vi "Drive Process.vi"(0 "error in":errorcluster) -> ()   [LabVIEW 2013]
uses:
  Drive Global Data.vi
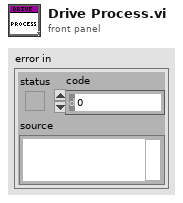
[diagram p1: front panel]
types:
  T1 = cluster{"Y":dbl, "X":dbl, "Left Encoder":dbl, "Right Encoder":dbl, "Slow Drive":bool}
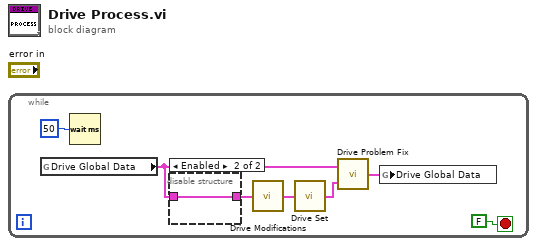
[diagram p0: block diagram]
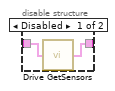
[diagram p2: hidden frame]
diagram:
  n1 = while {
    stop <- FALSE stop-if-true
    n2 = global read "Drive Global Data.vi" "Drive Global Data"() -> (w3:T1)
    n3 = Wait (ms)(milliseconds to wait=u32 50) -> ()  [unwired: 1 out]
    n4 = disable-structure shown="Enabled" {
      disable-tunnel: [w9 w10] -> w5
      disable-tunnel: w3 -> [w8 w10]
      frame Disabled {
        n5 = call "Drive GetSensors.vi"("Drive Global Data In"=w8) -> ("Drive Global Data Out"=w9:T1)
      }
      frame Enabled {
      }
    }
    n6 = call "Drive Modifications.vi"("Drive Global Data In"=w5) -> ("Drive Global Data Out"=w4:T1)
    n7 = call "Drive Set.vi"("Drive Global Data In"=w4) -> ("Drive Global Data Out"=w2:T1)
    n8 = call "Drive Problem Fix.vi"("Drive Global Data Modified"=w2, "Drive Global Data Original"=w3) -> ("Drive Global Data New"=w1:T1)
    n9 = global write "Drive Global Data.vi" "Drive Global Data"(w1) -> ()
  }
